vi "Unit test-Time series images save.vi"() -> ()   [LabVIEW 2017]
uses:
  Typedefs/Imaging Protocols enum.ctl
  Typedefs/Frame Size.ctl
  Typedefs/Logging queue element.ctl
  Typedefs/Acquired points count.ctl
panel:
  out "Loop time (ms) 2":u32
  out "Loop time (ms)":u32
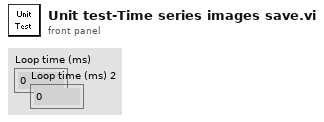
[diagram p1: front panel]
types:
  T1 = typedef "Logging queue element.ctl" = cluster{"Imaging Protocol":T2, "Number of Trials":u16, "Frame Size":T3, "# Averaged frames":u16, "Dwell time (us)":dbl, "Index of Z-plane":i32, "Timelapse?":bool, "Logging process is active":bool, "Speed logging enabled":bool, "tdms file ref":refnum<k34>, "path":path, "Trial Number":i32, "Expected # points acquired":bool, "Manually stopped":bool, "Ch0 data":u32[], "Ch1 data":u32[], "Ref Data":u32[], "Last trial":bool, "Ref Dwell time (us)":dbl, "# Ref Averaged frames":u16, "Ref X Length":u16, "Ref Y Length":u16, "Points acquired":T4}
  T2 = typedef "Imaging Protocols enum.ctl" = enum16{"AOL Z-Stack", "Motor Z Stack", "Functional Acquisition", "Single Plane Acquisition", "Volume Acquisition", "Live Imaging", "Live Plane Imaging", "Live Volume Imaging"}
  T3 = typedef "Frame Size.ctl" = u16
  T4 = typedef "Acquired points count.ctl" = cluster{"Ch0 last trial":u64, "Ch1 last trial":u64, "All trials":u64}
  T5 = typedef "Live imaging queue element.ctl" = cluster{"Red channel":T6, "Green channel":T6, "Ref Red channel":T6, "Ref Green channel":T6, "Mov cor":bool}
  T6 = typedef "IMAQ Image.ctl" = refnum<image>
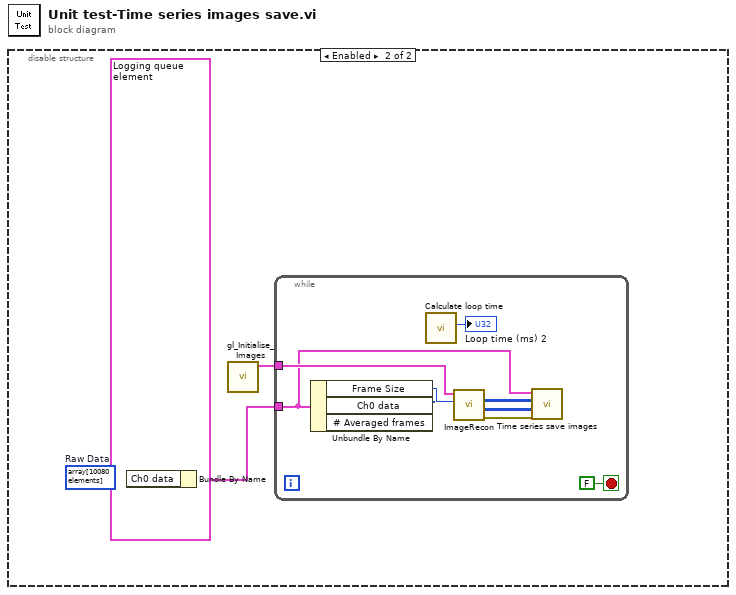
[diagram p0: block diagram]
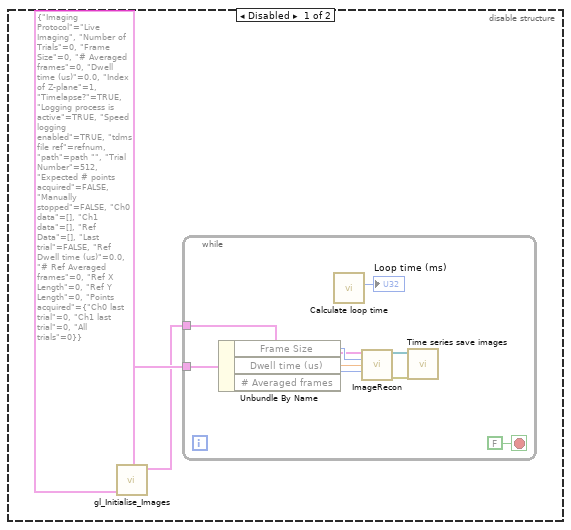
[diagram p2: hidden frame]
diagram:
  n1 = disable-structure shown="Enabled" {
    frame Disabled {
      n2 = call "gl_Initialise_Images.vi"() -> ("Live image refs"=w1:T5)  [unwired: 11 in]
      n3 = while {
        tunnel: T1 {"Imaging Protocol"=enum."Live Imaging", "Number of Trials"=0, "Frame Size"=0, "# Averaged frames"=0, "Dwell time (us)"=0.0, "Index of Z-plane"=1, "Timelapse?"=TRUE, "Logging process is active"=TRUE, "Speed logging enabled"=TRUE, "tdms file ref"=refnum, "path"=path "", "Trial Number"=512, "Expected # points acquired"=FALSE, "Manually stopped"=FALSE, "Ch0 data"=[], "Ch1 data"=[], "Ref Data"=[], "Last trial"=FALSE, "Ref Dwell time (us)"=0.0, "# Ref Averaged frames"=0, "Ref X Length"=0, "Ref Y Length"=0, "Points acquired"={"Ch0 last trial"=0, "Ch1 last trial"=0, "All trials"=0}} ("Logging queue element in") -> [w6]
        tunnel: w1 -> [w5]
        stop <- FALSE stop-if-true
        n4 = Unbundle By Name(w6) -> ("Frame Size"=w11:T3, "Dwell time (us)"=w10:dbl, "# Averaged frames"=w9:u16)
        n5 = call <userlib>:"Calculate loop time.vi"() -> ("Loop time (ms)"=→"Loop time (ms)":u32)  [unwired: 11 in]
        n6 = call "ImageRecon.vi"("Image Array (in)"=w5, "Frame Size"=w11, "dwelltime"=w10, "Waveforms"=w9) -> ("Image Array(out)"=w7:T6[], "Error Out"=w8:errorcluster)  [unwired: 8 in, 2 out]
        n7 = call "Time series save images.vi"("error in (no error)"=w8, "Logging queue element"=w7) -> ()  [unwired: 9 in, 1 out]
      }
    }
    frame Enabled {
      w14 = i32[] array[10080 elements]  # Raw Data
      n8 = Bundle By Name(cluster=T1 {"Imaging Protocol"=enum."Live Imaging", "Number of Trials"=0, "Frame Size"=512, "# Averaged frames"=1, "Dwell time (us)"=0.10000000149011612, "Index of Z-plane"=0, "Timelapse?"=FALSE, "Logging process is active"=TRUE, "Speed logging enabled"=FALSE, "tdms file ref"=refnum, "path"=path "", "Trial Number"=1, "Expected # points acquired"=FALSE, "Manually stopped"=TRUE, "Ch0 data"=array[10080 elements], "Ch1 data"=[], "Ref Data"=[], "Last trial"=FALSE, "Ref Dwell time (us)"=0.0, "# Ref Averaged frames"=0, "Ref X Length"=0, "Ref Y Length"=0, "Points acquired"={"Ch0 last trial"=0, "Ch1 last trial"=0, "All trials"=0}} ("Logging queue element in"), "Ch0 data"=w14) -> (w12:T1)
      n9 = call "gl_Initialise_Images.vi"() -> ("Live image refs"=w15:T5)  [unwired: 11 in]
      n10 = while {
        tunnel: w12 -> [w17]
        tunnel: w15 -> [w22]
        stop <- FALSE stop-if-true
        n11 = Unbundle By Name(w17) -> ("Frame Size"=w24:T3, "Ch0 data"=w16:u32[])  [unwired: 1 out]
        n12 = call <userlib>:"Calculate loop time.vi"() -> ("Loop time (ms)"=→"Loop time (ms) 2":u32)  [unwired: 11 in]
        n13 = call "ImageRecon.vi"("Data"=w16, "Frame Size"=w24, "Image Array (in)"=w22) -> ("Error Out"=w23:errorcluster, "Ch1-Green"=w18:i16[][], "Ch0-Red"=w19:i16[][])  [unwired: 5 in, 1 out]
        n14 = call "Time series save images.vi"("error in (no error)"=w23, "Ch1-Green"=w18, "Ch0-Red"=w19, "Logging queue element"=w17) -> ()  [unwired: 7 in, 1 out]
      }
    }
  }
